vi "Self Test Result.vi"(10 "VI Action":T1=enum."Read") -> (2 "Self Test Result":bool)   [LabVIEW 2010]
uses:
  status action.ctl
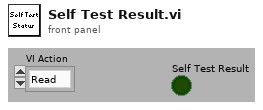
[diagram p1: front panel]
types:
  T1 = typedef "status action.ctl" = enum16{"Initialize", "Write", "Read"}
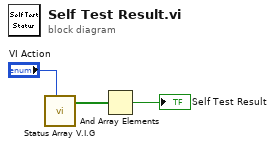
[diagram p0: block diagram]
diagram:
  n1 = call "Status Array V.I.G.vi"("VI Action"="VI Action") -> ("Array"=w2:bool[])  [unwired: 10 in]
  n2 = And Array Elements(Boolean array=w2) -> (logical AND=→"Self Test Result":bool)
